vi "Экзамен камень-ножницы-бумага.vi"() -> ()   [LabVIEW 2021]
panel:
  out "Счетчик Ваших побед":i32
  out "Счетчик побед компьютера":i32
  out "Вы":string
  out "String":string
  out "Компьютер":string
  out "Состояние":T1
  in  "Камень":bool
  in  "Бумага":bool
  in  "Ножницы":bool
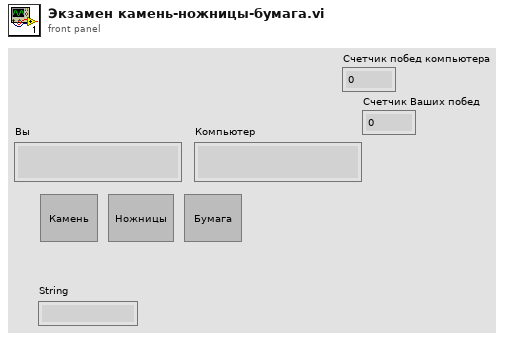
[diagram p1: front panel]
types:
  T1 = typedef "Экз1.ctl" = enum16{"Вы проиграли!", "Ничья!", "Вы победили!", "БумагаП-БумагаК", "НожницыП-БумагаК", "КаменьП-БумагаК", "БумагаП-НожницыК", "НожницыП-НожницыК", "КаменьП-НожницыК", "БумагаП-КаменьК", "НожницыП-КаменьК", "КаменьП-КаменьК", "Играем!"}
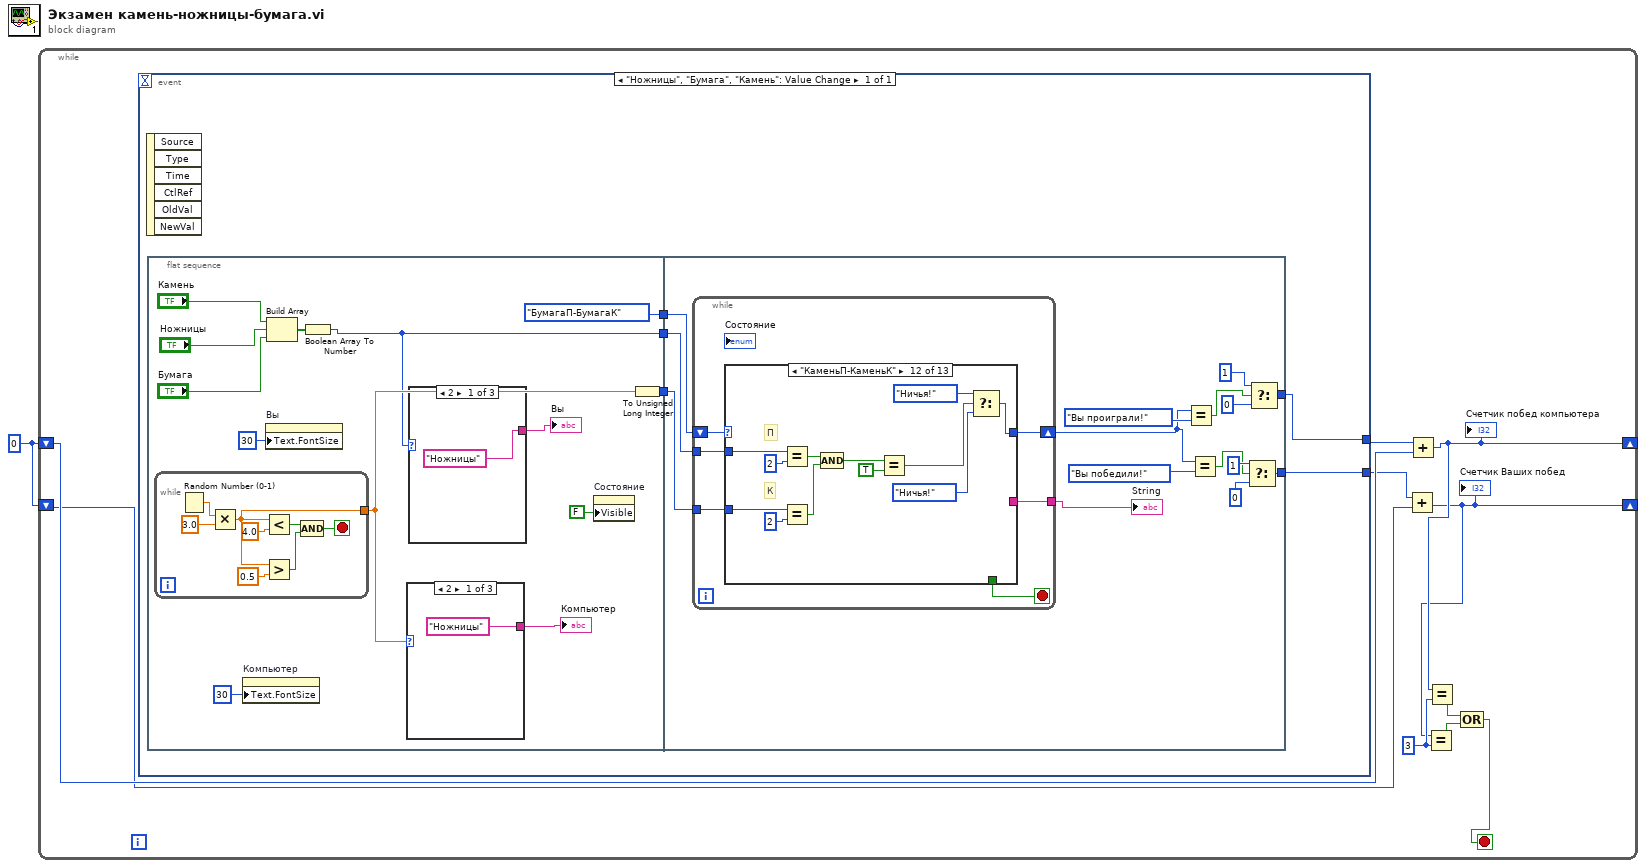
[diagram p0: block diagram]
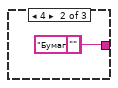
[diagram p2: hidden frame]
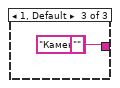
[diagram p3: hidden frame]
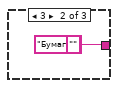
[diagram p4: hidden frame]
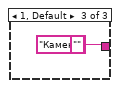
[diagram p5: hidden frame]
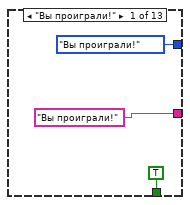
[diagram p6: hidden frame]
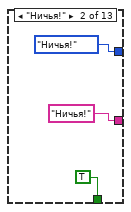
[diagram p7: hidden frame]
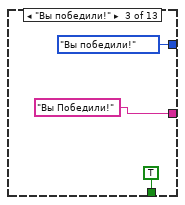
[diagram p8: hidden frame]
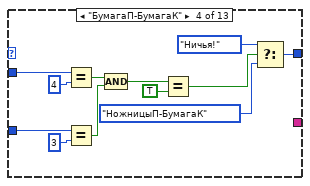
[diagram p9: hidden frame]
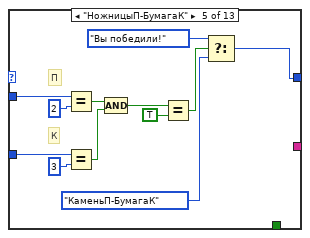
[diagram p10: hidden frame]
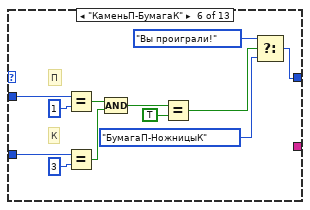
[diagram p11: hidden frame]
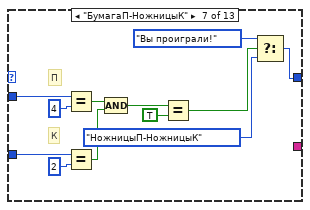
[diagram p12: hidden frame]
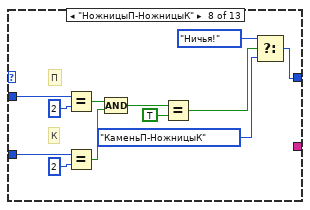
[diagram p13: hidden frame]
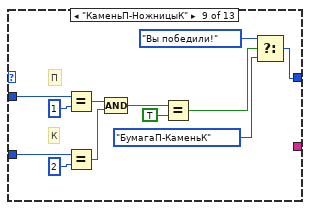
[diagram p14: hidden frame]
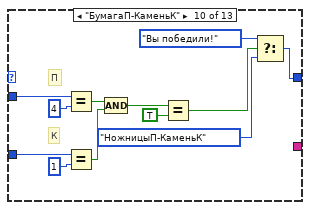
[diagram p15: hidden frame]
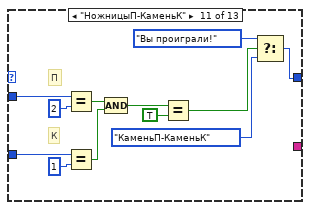
[diagram p16: hidden frame]
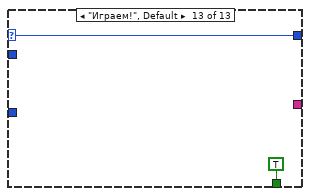
[diagram p17: hidden frame]
diagram:
  w1 = 0
  n1 = while {
    shift-right: [w3] -> _
    shift-left: w1 -> [w10]
    shift-right: [w2] -> _
    shift-left: w1 -> [w8]
    stop <- w6 stop-if-true
    w7 = 3 ("y")
    n2 = event shown="[0] \"Ножницы\", \"Бумага\", \"Камень\": Value Change" {
      selector: _ -> [_]
      dyn-events: _ -> [_]
      timeout: _ -> [_]
      tunnel: [w13] -> w11
      tunnel: [w12] -> w9
      event "Ножницы", "Бумага", "Камень": Value Change {
        n3 = event-data() -> ()  [unwired: 1 in, 6 out]
        n4 = flat-sequence {
          tunnel: [w25] -> w16
          tunnel: [w20] -> w15
          tunnel: [Экз1."БумагаП-БумагаК" ("Состояние")] -> w14
          tunnel: w16 -> [w58]
          tunnel: w15 -> [w57]
          tunnel: w14 -> [w56]
          tunnel: [w52] -> w13
          tunnel: [w44] -> w12
          frame #0 {
            n5 = while {
              tunnel: [w37] -> w22
              stop <- w33 stop-if-true
              n6 = Random Number (0-1)() -> (number: 0 to 1=w40:dbl)
              n7 = Multiply(x=w40, y=3.0) -> (x*y=w37:dbl)
              n8 = Less?(x=w37, y=4.0) -> (x < y?=w35:bool)
              n9 = Greater?(x=w37, y=0.5) -> (0:w34:bool)
              n10 = Compound Arithmetic op=AND(w35, w34) -> (w33:bool)
            }
            n11 = property on="Компьютер" class="Str"("Text.FontSize"=u32 30 ("Text.Font:Size")) -> ()  [unwired: 2 in, 2 out]
            n12 = property on="Вы" class="Str"("Text.FontSize"=u32 30 ("Text.Font:Size")) -> ()  [unwired: 2 in, 2 out]
            n13 = Build Array("Камень", "Ножницы", "Бумага") -> (w29:bool[])
            n14 = Boolean Array To Number(Boolean array=w29) -> (number=w20:u32)
            n15 = case shown="2" w22 {
              tunnel: ["Ножницы" ("Компьютер") "Бумага" ("Компьютер") "Камень" ("Компьютер")] -> w23
              frame 2 {
              }
              frame 3 {
                (unwired) "" ("Компьютер")
              }
              frame 1, Default {
                (unwired) "" ("Компьютер")
              }
            }
            "Компьютер" <- w23
            n16 = case shown="2" w20 {
              tunnel: ["Ножницы" ("Компьютер") "Бумага" ("Компьютер") "Камень" ("Компьютер")] -> w19
              frame 2 {
              }
              frame 4 {
                (unwired) "" ("Компьютер")
              }
              frame 1, Default {
                (unwired) "" ("Компьютер")
              }
            }
            "Вы" <- w19
            n17 = property on="Состояние" class="Enum (strict)"("Visible"=FALSE) -> ()  [unwired: 2 in, 2 out]
            n18 = To Unsigned Long Integer(number=w22) -> (unsigned 32bit integer=w25:u32)
          }
          frame #1 {
            n19 = while {
              tunnel: w58 -> [w62]
              tunnel: w57 -> [w63]
              shift-right: [w64] -> w49
              shift-left: w56 -> [w61]
              tunnel: [w59] -> w55
              stop <- w60 stop-if-true
              n20 = case shown="\"КаменьП-КаменьК\"" w61 {
                selector: w61 -> [_ _ _ _ _ _ _ _ _ _ _ _ w183]
                tunnel: w63 -> [_ _ _ w85 w97 w109 w121 w133 w145 w157 w169 w181 _]
                tunnel: w62 -> [_ _ _ w83 w95 w107 w119 w131 w143 w155 w167 w179 _]
                tunnel: [Экз1."Вы проиграли!" ("Состояние") Экз1."Ничья!" ("Состояние") Экз1."Вы победили!" ("Состояние") w74 w89 w101 w113 w125 w137 w149 w161 w173 w183] -> w64
                tunnel: [TRUE TRUE TRUE _ _ _ _ _ _ _ _ _ TRUE] -> w60
                tunnel: ["Вы проиграли!" ("String") "Ничья!" ("String") "Вы Победили!" ("String") _ _ _ _ _ _ _ _ _ _] -> w59
                frame "Вы проиграли!" {
                }
                frame "Ничья!" {
                }
                frame "Вы победили!" {
                }
                frame "БумагаП-БумагаК" {
                  n21 = Equal?(x=w85, y=u32 4) -> (x = y?=w81:bool)
                  n22 = Equal?(x=w83, y=u32 3) -> (x = y?=w80:bool)
                  n23 = Compound Arithmetic op=AND(w81, w80) -> (w79:bool)
                  n24 = Equal?(x=w79, y=TRUE) -> (x = y?=w77:bool)
                  n25 = Select(t=Экз1."Ничья!" ("Состояние"), s=w77, f=Экз1."НожницыП-БумагаК" ("Состояние")) -> (s? t:f=w74:T1)
                }
                frame "НожницыП-БумагаК" {
                  # "К"
                  # "П"
                  n26 = Equal?(x=w97, y=u32 2) -> (x = y?=w91:bool)
                  n27 = Equal?(x=w95, y=u32 3) -> (x = y?=w90:bool)
                  n28 = Compound Arithmetic op=AND(w91, w90) -> (w93:bool)
                  n29 = Equal?(x=w93, y=TRUE) -> (x = y?=w86:bool)
                  n30 = Select(t=Экз1."Вы победили!" ("Состояние"), s=w86, f=Экз1."КаменьП-БумагаК" ("Состояние")) -> (s? t:f=w89:T1)
                }
                frame "КаменьП-БумагаК" {
                  # "К"
                  # "П"
                  n31 = Equal?(x=w109, y=u32 1) -> (x = y?=w103:bool)
                  n32 = Equal?(x=w107, y=u32 3) -> (x = y?=w102:bool)
                  n33 = Compound Arithmetic op=AND(w103, w102) -> (w105:bool)
                  n34 = Equal?(x=w105, y=TRUE) -> (x = y?=w98:bool)
                  n35 = Select(t=Экз1."Вы проиграли!" ("Состояние"), s=w98, f=Экз1."БумагаП-НожницыК" ("Состояние")) -> (s? t:f=w101:T1)
                }
                frame "БумагаП-НожницыК" {
                  # "К"
                  # "П"
                  n36 = Equal?(x=w121, y=u32 4) -> (x = y?=w115:bool)
                  n37 = Equal?(x=w119, y=u32 2) -> (x = y?=w114:bool)
                  n38 = Compound Arithmetic op=AND(w115, w114) -> (w117:bool)
                  n39 = Equal?(x=w117, y=TRUE) -> (x = y?=w110:bool)
                  n40 = Select(t=Экз1."Вы проиграли!" ("Состояние"), s=w110, f=Экз1."НожницыП-НожницыК" ("Состояние")) -> (s? t:f=w113:T1)
                }
                frame "НожницыП-НожницыК" {
                  # "К"
                  # "П"
                  n41 = Equal?(x=w133, y=u32 2) -> (x = y?=w127:bool)
                  n42 = Equal?(x=w131, y=u32 2) -> (x = y?=w126:bool)
                  n43 = Compound Arithmetic op=AND(w127, w126) -> (w129:bool)
                  n44 = Equal?(x=w129, y=TRUE) -> (x = y?=w122:bool)
                  n45 = Select(t=Экз1."Ничья!" ("Состояние"), s=w122, f=Экз1."КаменьП-НожницыК" ("Состояние")) -> (s? t:f=w125:T1)
                }
                frame "КаменьП-НожницыК" {
                  # "К"
                  # "П"
                  n46 = Equal?(x=w145, y=u32 1) -> (x = y?=w139:bool)
                  n47 = Equal?(x=w143, y=u32 2) -> (x = y?=w138:bool)
                  n48 = Compound Arithmetic op=AND(w139, w138) -> (w141:bool)
                  n49 = Equal?(x=w141, y=TRUE) -> (x = y?=w134:bool)
                  n50 = Select(t=Экз1."Вы победили!" ("Состояние"), s=w134, f=Экз1."БумагаП-КаменьК" ("Состояние")) -> (s? t:f=w137:T1)
                }
                frame "БумагаП-КаменьК" {
                  # "К"
                  # "П"
                  n51 = Equal?(x=w157, y=u32 4) -> (x = y?=w151:bool)
                  n52 = Equal?(x=w155, y=u32 1) -> (x = y?=w150:bool)
                  n53 = Compound Arithmetic op=AND(w151, w150) -> (w153:bool)
                  n54 = Equal?(x=w153, y=TRUE) -> (x = y?=w146:bool)
                  n55 = Select(t=Экз1."Вы победили!" ("Состояние"), s=w146, f=Экз1."НожницыП-КаменьК" ("Состояние")) -> (s? t:f=w149:T1)
                }
                frame "НожницыП-КаменьК" {
                  # "К"
                  # "П"
                  n56 = Equal?(x=w169, y=u32 2) -> (x = y?=w163:bool)
                  n57 = Equal?(x=w167, y=u32 1) -> (x = y?=w162:bool)
                  n58 = Compound Arithmetic op=AND(w163, w162) -> (w165:bool)
                  n59 = Equal?(x=w165, y=TRUE) -> (x = y?=w158:bool)
                  n60 = Select(t=Экз1."Вы проиграли!" ("Состояние"), s=w158, f=Экз1."КаменьП-КаменьК" ("Состояние")) -> (s? t:f=w161:T1)
                }
                frame "КаменьП-КаменьК" {
                  # "К"
                  # "П"
                  n61 = Equal?(x=w181, y=u32 2) -> (x = y?=w175:bool)
                  n62 = Equal?(x=w179, y=u32 2) -> (x = y?=w174:bool)
                  n63 = Compound Arithmetic op=AND(w175, w174) -> (w177:bool)
                  n64 = Equal?(x=w177, y=TRUE) -> (x = y?=w170:bool)
                  n65 = Select(t=Экз1."Ничья!" ("Состояние"), s=w170, f=Экз1."Ничья!" ("Состояние")) -> (s? t:f=w173:T1)
                }
                frame "Играем!", Default {
                }
              }
            }
            "String" <- w55
            n66 = Equal?(x=w49, y=Экз1."Вы проиграли!" ("Состояние")) -> (x = y?=w45:bool)
            n67 = Equal?(x=w49, y=Экз1."Вы победили!" ("Состояние")) -> (x = y?=w46:bool)
            n68 = Select(t=1, s=w46, f=0) -> (s? t:f=w44:i32)
            n69 = Select(t=1, s=w45, f=0) -> (s? t:f=w52:i32)
          }
        }
      }
    }
    n70 = Add(x=w9, y=w8) -> (x+y=w2:i32)
    "Счетчик Ваших побед" <- w2
    n71 = Add(x=w11, y=w10) -> (x+y=w3:i32)
    "Счетчик побед компьютера" <- w3
    n72 = Equal?(x=w2, y=w7) -> (x = y?=w4:bool)
    n73 = Equal?(x=w3, y=w7) -> (x = y?=w5:bool)
    n74 = Compound Arithmetic op=OR(w5, w4) -> (w6:bool)
  }
